vi "Read.Data.Detect.vi"(5 "length":i32=-1, 7 "index":i32, 8 "error in":errorcluster, 10 "timeout ms":i32, 11 "Ref":T1) -> (0 "error out":errorcluster, 1 "Timeout?":bool, 2 "Values":dbl[](array[numeric]), 3 "Detect?":bool[](array[boolean]))   [LabVIEW 2023, in "Plugin Data Access Engine.lvlib" / "Plugin Data Access Engine.lvclass"]
uses:
  Plugin Data Access Engine.lvclass
  Types/Read.DVR.ctl
  Access Type Classes/Read/Read.lvclass
  Access Type Classes/Read/Read.lvclass/Read.ctl
  Plugin Data Access Engine.lvclass/Plugin Data Access Engine.ctl
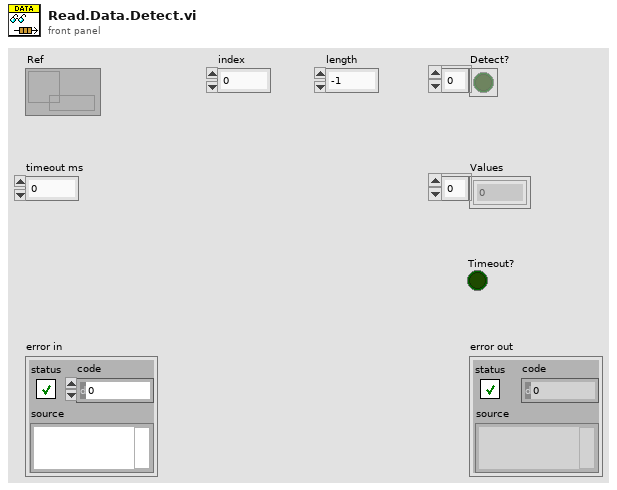
[diagram p1: front panel]
types:
  T1 = typedef "Plugin Data Access Engine.lvlib/Plugin Data Access Engine.lvclass/Read.DVR.ctl" = refnum<data-value>
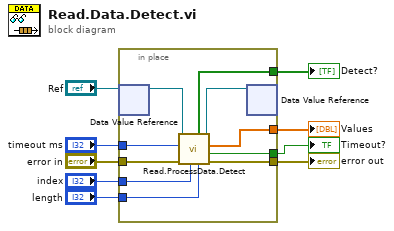
[diagram p0: block diagram]
diagram:
  n1 = in-place {
    in-place-border: "error in" -> [w19]
    in-place-border: [w18] -> w8
    in-place-border: [w15] -> w6
    in-place-border: "timeout ms" -> [w14]
    in-place-border: [w13] -> w4
    in-place-border: "index" -> [w12]
    in-place-border: "length" -> [w11]
    in-place-border: [w10] -> w1
    n2 = in-place-dvr #1("Ref") -> (w17:refnum<class "Read.lvclass">)  [unwired: 1 out]
    n3 = call "Read.ProcessData.Detect.vi"("length"=w11, "index"=w12, "error in"=w19, "timeout ms"=w14, "Read in"=w17) -> ("error out"=w18:errorcluster, "Timeout?"=w13:bool, "Data"=w15:dbl[], "Read out"=w16:refnum<class "Read.lvclass">, "Detect?"=w10:bool[])  [unwired: 2 in]
    n4 = in-place-dvr #1(w16) -> ()  [unwired: 2 out]
  }
  "error out" <- w8
  "Values" <- w6
  "Timeout?" <- w4
  "Detect?" <- w1
